vi "Time Estimate.vi"(8 "error in (no error)":errorcluster, 9 "expmode":i32, 10 "scantype":T1(ring), 11 "Pulse Gen Scan.lvclass":refnum<class "Pulse Gen Scan.lvclass">) -> (0 "error out":errorcluster, 1 "Time Estimate":string, 2 "time":dbl[unit], 3 "Pulse Gen Scan.lvclass":refnum<class "Pulse Gen Scan.lvclass">)   [LabVIEW 2012, in "Pulse Gen Scan.lvclass"]
uses:
  Pulse Gen Scan.lvclass
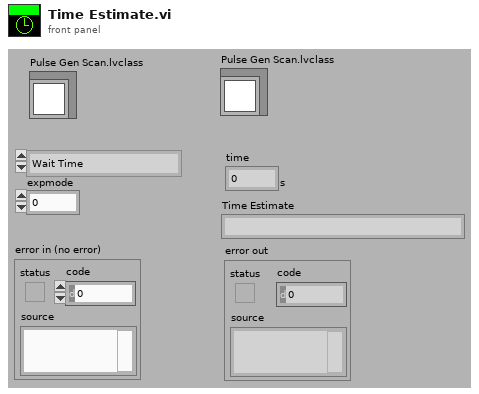
[diagram p1: front panel]
types:
  T1 = enum16{"Wait Time", "Pulse Width", "Wavelength", "Magnetic Field", "rf Scan"}
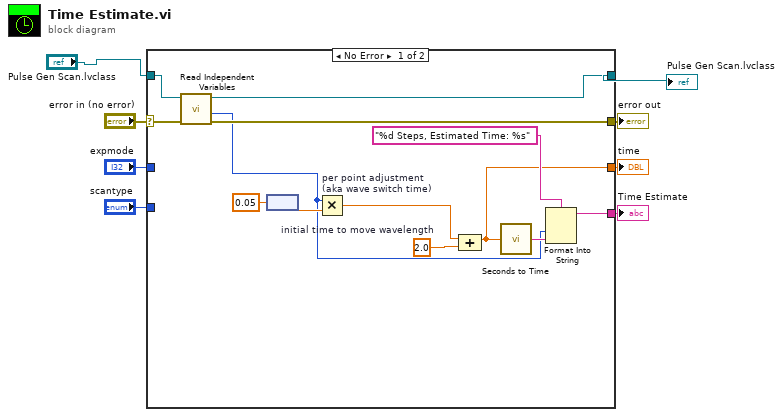
[diagram p0: block diagram]
diagram:
  n1 = case shown="No Error" "error in (no error)" {
    selector: "error in (no error)" -> [w18 w22]
    tunnel: [w15 _] -> w4
    tunnel: "expmode" -> [_ _]
    tunnel: "scantype" -> [_ _]
    tunnel: [w19 w23] -> w2
    tunnel: "Pulse Gen Scan.lvclass" -> [w20 w23]
    tunnel: [w21 w22] -> w6
    tunnel: [w10 _] -> w1
    frame No Error {
      w13 = dbl[unit] 2.0  # initial time to move wavelength
      n2 = call-dynamic "Read Independent Variables.vi"("error in (no error)"=w18, "Scanner.lvclass in"=w20) -> ("error out"=w21:errorcluster, "size"=w9:i32, "Scanner.lvclass out"=w19:refnum<class "Pulse Gen Scan.lvclass">)  [unwired: 7 out]
      n3 = node(0.05) -> (w11:dbl[unit])
      n4 = Multiply "per point adjustment\n(aka wave switch time)"(x=w9, y=w11) -> (x*y=w14:dbl[unit])
      n5 = Compound Arithmetic op=ADD(w14, w13) -> (w10:dbl[unit])
      n6 = call "Seconds to Time.vi"("Seconds"=w10) -> ("Time"=w16:string)
      n7 = Format Into String(format string="%d Steps, Estimated Time: %s", w9, w16) -> (resulting string=w15:string)  [unwired: 2 in, 1 out]
    }
    frame Error {
    }
  }
  "time" <- w1
  "error out" <- w6
  "Time Estimate" <- w4
  "Pulse Gen Scan.lvclass" <- w2
